vi "Configure Measurement.vi"(8 "error in (no error)":errorcluster, 10 "Function (0: Cp-D)":T1, 11 "Agilent 428x in":refnum<class "Agilent 428x.lvclass">) -> (0 "error out":errorcluster, 3 "Agilent 428x out":refnum<class "Agilent 428x.lvclass">)   [LabVIEW 2020, in "Agilent 428x.lvclass"]
uses:
  Agilent 428x.lvclass
  C:/Sandbox/Git_Sandbox/WiSpry Test Framework source code (LV20)/WiSpry Test Framework/Instruments/Instrument.lvclass
  Controls/Function.ctl
  Instrument.lvclass/Instrument.ctl
  Instrument.lvclass
  <instrlib>/Agilent 428X Series/Agilent 428X Series.lvlib
  LCR Meter.lvclass
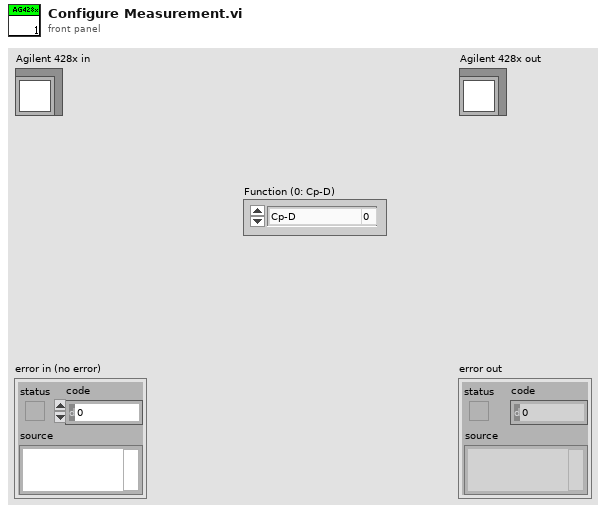
[diagram p1: front panel]
types:
  T1 = typedef "LCR Meter.lvclass/Function.ctl" = enum16{"Cp-D", "Cp-Q", "Cp-G", "Cp-Rp", "Cs-D", "Cs-Q", "Cs-Rs", "Lp-D", "Lp-Q", "Lp-G", "Lp-Rp", "Lp-Rdc", "Ls-D", "Ls-Q", "Ls-Rs", "Ls-Rdc", "R-X", "Z-thd", "Z-thr", "G-B", "Y-thd", "Y-thr", "Vdc-Idc"}
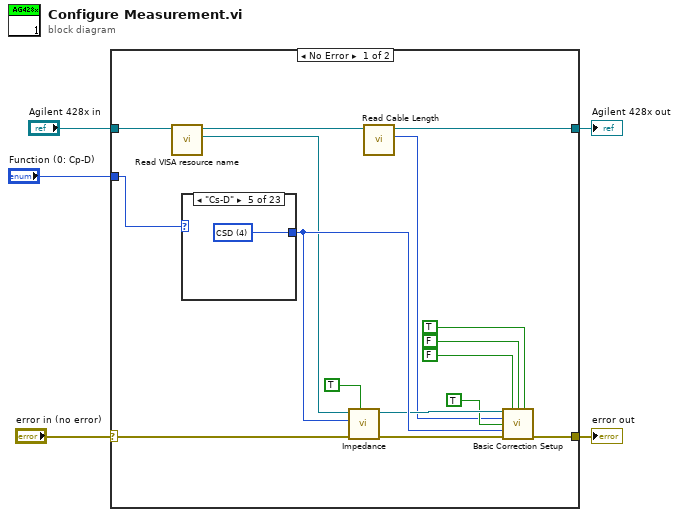
[diagram p0: block diagram]
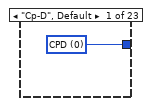
[diagram p2: hidden frame]
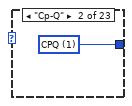
[diagram p3: hidden frame]
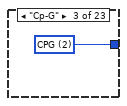
[diagram p4: hidden frame]
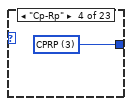
[diagram p5: hidden frame]
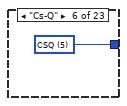
[diagram p6: hidden frame]
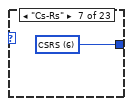
[diagram p7: hidden frame]
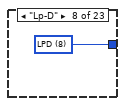
[diagram p8: hidden frame]
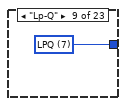
[diagram p9: hidden frame]
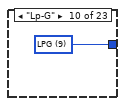
[diagram p10: hidden frame]
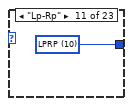
[diagram p11: hidden frame]
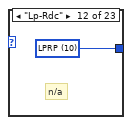
[diagram p12: hidden frame]
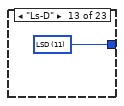
[diagram p13: hidden frame]
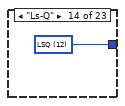
[diagram p14: hidden frame]
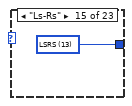
[diagram p15: hidden frame]
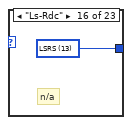
[diagram p16: hidden frame]
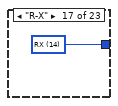
[diagram p17: hidden frame]
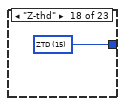
[diagram p18: hidden frame]
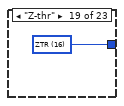
[diagram p19: hidden frame]
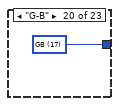
[diagram p20: hidden frame]
diagram:
  n1 = case shown="No Error" "error in (no error)" {
    selector: "error in (no error)" -> [w17 w46]
    tunnel: [w20 w46] -> w5
    tunnel: [w7 w45] -> w4
    tunnel: "Agilent 428x in" -> [w21 w45]
    tunnel: "Function (0: Cp-D)" -> [w19 _]
    frame No Error {
      n2 = call "Read VISA resource name.vi"("Instrument in"=w21) -> ("VISA resource name"=w15:refnum<visa-resource-name>, "Instrument out"=w8:refnum<class "Agilent 428x.lvclass">)  [unwired: 9 in]
      n3 = case shown="\"Cs-D\"" w19 {
        tunnel: [w22 w23 w24 w25 w26 w27 w28 w29 w30 w31 w32 w33 w34 w35 w36 w37 w38 w39 w40 w41 w42 w43 w44] -> w18
        frame "Cp-D", Default {
          w22 = u32 0 items=["CPD", "CPQ", "CPG", "CPRP", "CSD", "CSQ", "CSRS", "LPQ", "LPD", "LPG", "LPRP", "LSD", "LSQ", "LSRS", "RX", "ZTD", "ZTR", "GB", "YTD", "YTR"] ("Load Type (0: CPD)")
        }
        frame "Cp-Q" {
          w23 = u32 1 items=["CPD", "CPQ", "CPG", "CPRP", "CSD", "CSQ", "CSRS", "LPQ", "LPD", "LPG", "LPRP", "LSD", "LSQ", "LSRS", "RX", "ZTD", "ZTR", "GB", "YTD", "YTR"] ("Load Type (0: CPD)")
        }
        frame "Cp-G" {
          w24 = u32 2 items=["CPD", "CPQ", "CPG", "CPRP", "CSD", "CSQ", "CSRS", "LPQ", "LPD", "LPG", "LPRP", "LSD", "LSQ", "LSRS", "RX", "ZTD", "ZTR", "GB", "YTD", "YTR"] ("Load Type (0: CPD)")
        }
        frame "Cp-Rp" {
          w25 = u32 3 items=["CPD", "CPQ", "CPG", "CPRP", "CSD", "CSQ", "CSRS", "LPQ", "LPD", "LPG", "LPRP", "LSD", "LSQ", "LSRS", "RX", "ZTD", "ZTR", "GB", "YTD", "YTR"] ("Load Type (0: CPD)")
        }
        frame "Cs-D" {
          w26 = u32 4 items=["CPD", "CPQ", "CPG", "CPRP", "CSD", "CSQ", "CSRS", "LPQ", "LPD", "LPG", "LPRP", "LSD", "LSQ", "LSRS", "RX", "ZTD", "ZTR", "GB", "YTD", "YTR"] ("Load Type (0: CPD)")
        }
        frame "Cs-Q" {
          w27 = u32 5 items=["CPD", "CPQ", "CPG", "CPRP", "CSD", "CSQ", "CSRS", "LPQ", "LPD", "LPG", "LPRP", "LSD", "LSQ", "LSRS", "RX", "ZTD", "ZTR", "GB", "YTD", "YTR"] ("Load Type (0: CPD)")
        }
        frame "Cs-Rs" {
          w28 = u32 6 items=["CPD", "CPQ", "CPG", "CPRP", "CSD", "CSQ", "CSRS", "LPQ", "LPD", "LPG", "LPRP", "LSD", "LSQ", "LSRS", "RX", "ZTD", "ZTR", "GB", "YTD", "YTR"] ("Load Type (0: CPD)")
        }
        frame "Lp-D" {
          w29 = u32 8 items=["CPD", "CPQ", "CPG", "CPRP", "CSD", "CSQ", "CSRS", "LPQ", "LPD", "LPG", "LPRP", "LSD", "LSQ", "LSRS", "RX", "ZTD", "ZTR", "GB", "YTD", "YTR"] ("Load Type (0: CPD)")
        }
        frame "Lp-Q" {
          w30 = u32 7 items=["CPD", "CPQ", "CPG", "CPRP", "CSD", "CSQ", "CSRS", "LPQ", "LPD", "LPG", "LPRP", "LSD", "LSQ", "LSRS", "RX", "ZTD", "ZTR", "GB", "YTD", "YTR"] ("Load Type (0: CPD)")
        }
        frame "Lp-G" {
          w31 = u32 9 items=["CPD", "CPQ", "CPG", "CPRP", "CSD", "CSQ", "CSRS", "LPQ", "LPD", "LPG", "LPRP", "LSD", "LSQ", "LSRS", "RX", "ZTD", "ZTR", "GB", "YTD", "YTR"] ("Load Type (0: CPD)")
        }
        frame "Lp-Rp" {
          w32 = u32 10 items=["CPD", "CPQ", "CPG", "CPRP", "CSD", "CSQ", "CSRS", "LPQ", "LPD", "LPG", "LPRP", "LSD", "LSQ", "LSRS", "RX", "ZTD", "ZTR", "GB", "YTD", "YTR"] ("Load Type (0: CPD)")
        }
        frame "Lp-Rdc" {
          w33 = u32 10 items=["CPD", "CPQ", "CPG", "CPRP", "CSD", "CSQ", "CSRS", "LPQ", "LPD", "LPG", "LPRP", "LSD", "LSQ", "LSRS", "RX", "ZTD", "ZTR", "GB", "YTD", "YTR"] ("Load Type (0: CPD)")
          # "n/a"
        }
        frame "Ls-D" {
          w34 = u32 11 items=["CPD", "CPQ", "CPG", "CPRP", "CSD", "CSQ", "CSRS", "LPQ", "LPD", "LPG", "LPRP", "LSD", "LSQ", "LSRS", "RX", "ZTD", "ZTR", "GB", "YTD", "YTR"] ("Load Type (0: CPD)")
        }
        frame "Ls-Q" {
          w35 = u32 12 items=["CPD", "CPQ", "CPG", "CPRP", "CSD", "CSQ", "CSRS", "LPQ", "LPD", "LPG", "LPRP", "LSD", "LSQ", "LSRS", "RX", "ZTD", "ZTR", "GB", "YTD", "YTR"] ("Load Type (0: CPD)")
        }
        frame "Ls-Rs" {
          w36 = u32 13 items=["CPD", "CPQ", "CPG", "CPRP", "CSD", "CSQ", "CSRS", "LPQ", "LPD", "LPG", "LPRP", "LSD", "LSQ", "LSRS", "RX", "ZTD", "ZTR", "GB", "YTD", "YTR"] ("Load Type (0: CPD)")
        }
        frame "Ls-Rdc" {
          w37 = u32 13 items=["CPD", "CPQ", "CPG", "CPRP", "CSD", "CSQ", "CSRS", "LPQ", "LPD", "LPG", "LPRP", "LSD", "LSQ", "LSRS", "RX", "ZTD", "ZTR", "GB", "YTD", "YTR"] ("Load Type (0: CPD)")
          # "n/a"
        }
        frame "R-X" {
          w38 = u32 14 items=["CPD", "CPQ", "CPG", "CPRP", "CSD", "CSQ", "CSRS", "LPQ", "LPD", "LPG", "LPRP", "LSD", "LSQ", "LSRS", "RX", "ZTD", "ZTR", "GB", "YTD", "YTR"] ("Load Type (0: CPD)")
        }
        frame "Z-thd" {
          w39 = u32 15 items=["CPD", "CPQ", "CPG", "CPRP", "CSD", "CSQ", "CSRS", "LPQ", "LPD", "LPG", "LPRP", "LSD", "LSQ", "LSRS", "RX", "ZTD", "ZTR", "GB", "YTD", "YTR"] ("Load Type (0: CPD)")
        }
        frame "Z-thr" {
          w40 = u32 16 items=["CPD", "CPQ", "CPG", "CPRP", "CSD", "CSQ", "CSRS", "LPQ", "LPD", "LPG", "LPRP", "LSD", "LSQ", "LSRS", "RX", "ZTD", "ZTR", "GB", "YTD", "YTR"] ("Load Type (0: CPD)")
        }
        frame "G-B" {
          w41 = u32 17 items=["CPD", "CPQ", "CPG", "CPRP", "CSD", "CSQ", "CSRS", "LPQ", "LPD", "LPG", "LPRP", "LSD", "LSQ", "LSRS", "RX", "ZTD", "ZTR", "GB", "YTD", "YTR"] ("Load Type (0: CPD)")
        }
        frame "Y-thd" {
          w42 = u32 18 items=["CPD", "CPQ", "CPG", "CPRP", "CSD", "CSQ", "CSRS", "LPQ", "LPD", "LPG", "LPRP", "LSD", "LSQ", "LSRS", "RX", "ZTD", "ZTR", "GB", "YTD", "YTR"] ("Load Type (0: CPD)")
        }
        frame "Y-thr" {
          w43 = u32 19 items=["CPD", "CPQ", "CPG", "CPRP", "CSD", "CSQ", "CSRS", "LPQ", "LPD", "LPG", "LPRP", "LSD", "LSQ", "LSRS", "RX", "ZTD", "ZTR", "GB", "YTD", "YTR"] ("Load Type (0: CPD)")
        }
        frame "Vdc-Idc" {
          w44 = u32 2 items=["CPD", "CPQ", "CPG", "CPRP", "CSD", "CSQ", "CSRS", "LPQ", "LPD", "LPG", "LPRP", "LSD", "LSQ", "LSRS", "RX", "ZTD", "ZTR", "GB", "YTD", "YTR"] ("Load Type (0: CPD)")
          # "n/a"
        }
      }
      n4 = call <instrlib>:"Impedance.vi"("Auto Range (F: Off)"=TRUE, "error in (no error)"=w17, "Imp Type (0: CPD)"=w18, "VISA resource name"=w15) -> ("error out"=w16:errorcluster, "VISA resource name out"=w14:refnum<visa-resource-name>)  [unwired: 6 in]
      n5 = call-dynamic "Read Cable Length.vi"("Agilent 428x in"=w8) -> ("Cable Length (0: 0 m)"=w6:u32, "Agilent 428x out"=w7:refnum<class "Agilent 428x.lvclass">)  [unwired: 8 in, 1 out]
      n6 = call <instrlib>:"Basic Correction Setup.vi"("VISA resource name"=w14, "Load Corr  (F: Off)"=FALSE ("Short Corr (T: On)"), "Short Corr (T: On)"=FALSE, "Open Corr  (F: Off)"=TRUE, "Cable Length (0: 4 m)"=w6, "Corr Method (T: Single)"=TRUE, "Load Type (0: CPD)"=w18, "error in (no error)"=w16) -> ("error out"=w20:errorcluster)  [unwired: 5 in, 2 out]
    }
    frame Error {
    }
  }
  "error out" <- w5
  "Agilent 428x out" <- w4
